vi "tsa_AR F-B.vi"(9 "method":enum16{"FB", "Cov", "YuleWalker"}(ring), 10 "AR order":i32, 11 "response signal":dbl[](array[numeric]) format="%.2f") -> (0 "error":i32, 1 "noise variance":dbl format="%.10e", 2 "noise":dbl[](array[numeric]) format="%.2f", 3 "AR coefficents":dbl[](array[numeric]) format="%.2f", 4 "sita^2":dbl)   [LabVIEW 2024, in "NI_AALPro.lvlib"]
uses:
  NI_AALPro.lvlib
  Real Dot Product.vi
  Real PseudoInverse Matrix.vi
  A x Vector.vi
  NI_AALBase.lvlib
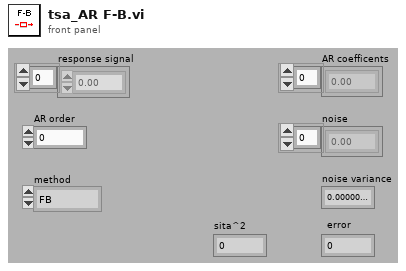
[diagram p1: front panel]
types:
  T1 = typedef "NI_Matrix.lvlib/RealMatrix.ctl" = dbl[][]
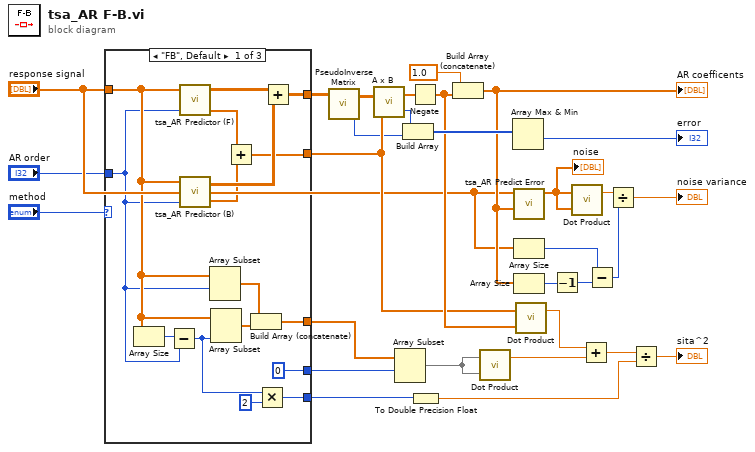
[diagram p0: block diagram]
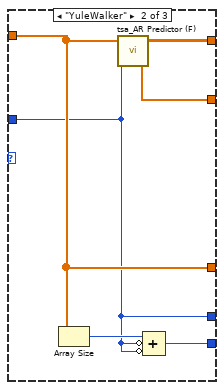
[diagram p2: hidden frame]
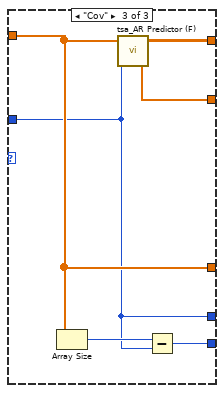
[diagram p3: hidden frame]
diagram:
  n1 = case shown="\"FB\", Default" "method" {
    tunnel: "response signal" -> [w40 w49 w56]
    tunnel: "AR order" -> [w39 w47 w54]
    tunnel: [w45 w52 w58] -> w3
    tunnel: [w43 w51 w57] -> w6
    tunnel: [0 ("AR order") w47 w54] -> w10
    tunnel: [w36 w49 w56] -> w9
    tunnel: [w32 w48 w53] -> w8
    frame "FB", Default {
      n2 = Array Size(array=w40) -> (size(s)=w35:i32)
      n3 = Subtract(x=w35, y=w39) -> (x-y=w31:i32)
      n4 = call "tsa_AR Predictor (F).vi"("Response signal"=w40, "order"=w39) -> ("R Matrix"=w42:dbl[][], "F Vector"=w41:dbl[])  [unwired: 4 in]
      n5 = call "tsa_AR Predictor (B).vi"("Response signal"=w40, "order"=w39) -> ("Backward Matrix"=w46:dbl[][], "Backward Vector"=w44:dbl[])  [unwired: 3 in]
      n6 = Array Subset(array=w40, index=w39) -> (w38:dbl[])  [unwired: 1 in]
      n7 = Array Subset(array=w40, length=w31) -> (w37:dbl[])  [unwired: 1 in]
      n8 = Add(x=w41, y=w44) -> (x+y=w43:dbl[])
      n9 = Build Array (concatenate)(w38, w37) -> (w36:dbl[])
      n10 = Multiply(x=w31, y=2) -> (x*y=w32:i32)
      n11 = Add(x=w42, y=w46) -> (x+y=w45:dbl[][])
    }
    frame "YuleWalker" {
      n12 = Array Size(array=w49) -> (size(s)=w50:i32)
      n13 = call "tsa_AR Predictor (F).vi"("Response signal"=w49, "order"=w47) -> ("R Matrix"=w52:dbl[][], "F Vector"=w51:dbl[])  [unwired: 4 in]
      n14 = Compound Arithmetic op=ADD(w50, invert w47, invert w47) -> (w48:i32)
    }
    frame "Cov" {
      n15 = Array Size(array=w56) -> (size(s)=w55:i32)
      n16 = call "tsa_AR Predictor (F).vi"("Response signal"=w56, "order"=w54) -> ("R Matrix"=w58:dbl[][], "F Vector"=w57:dbl[])  [unwired: 4 in]
      n17 = Subtract(x=w55, y=w54) -> (x-y=w53:i32)
    }
  }
  n18 = call-poly "PseudoInverse Matrix.vi"("Input Matrix"=w3) -> ("error"=w1:i32, "PseudoInverse Matrix"=w2:T1)  [unwired: 1 in]
  n19 = call-poly "A x B.vi"("Vector"=w6, "A"=w2) -> ("error"=w21:i32, "A x Vector"=w29:dbl[])
  n20 = Array Subset(array=w9, index=w10) -> (w16:dbl[])  [unwired: 1 in]
  n21 = Build Array(w21, w1) -> (w20:i32[])
  n22 = Negate(x=w29) -> (-x=w7:dbl[])
  n23 = To Double Precision Float(number=w8) -> (double precision float=w14:dbl)
  n24 = Build Array (concatenate)(1.0, w7) -> (w13:dbl[])
  "AR coefficents" <- w13
  n25 = call-poly "Dot Product.vi"("Y Vector"=w16, "X Vector"=w16) -> ("X * Y"=w17:dbl)  [unwired: 1 out]
  n26 = Array Max & Min(array=w20) -> (min value=→"error":i32)  [unwired: 3 out]
  n27 = call "tsa_AR Predict Error.vi"("Xt"="response signal", "AR coefficents"=w13) -> ("error"=w18:dbl[])  [unwired: 7 in, 1 out]
  "noise" <- w18
  n28 = Array Size(array="response signal") -> (size(s)=w25:i32)
  n29 = Array Size(array=w13) -> (size(s)=w26:i32)
  n30 = call-poly "Dot Product.vi"("Y Vector"=w7, "X Vector"=w6) -> ("X * Y"=w12:dbl)  [unwired: 1 out]
  n31 = Decrement(x=w26) -> (x-1=w24:i32)
  n32 = call-poly "Dot Product.vi"("Y Vector"=w18, "X Vector"=w18) -> ("X * Y"=w27:dbl)  [unwired: 1 out]
  n33 = Add(x=w12, y=w17) -> (x+y=w15:dbl)
  n34 = Subtract(x=w25, y=w24) -> (x-y=w23:i32)
  n35 = Divide(x=w27, y=w23) -> (x/y=→"noise variance":dbl)
  n36 = Divide(x=w15, y=w14) -> (x/y=→"sita^2":dbl)
